vi "test capture.vi"() -> ()   [LabVIEW 2014]
uses:
  <vilib>/Utility/inputDevices.llb/joystickAcquire.vi
  <vilib>/Utility/inputDevices.llb/closeJoystick.vi
panel:
  in  "Stop All":bool=TRUE
  out "button 4":bool
  out "button 3":bool
  in  "Motor Cruise Param":T1={"X Acc (mm/s^2)"=0.3, "X Vmax (mm/s)"=0.3, "Y Acc (mm/s^2)"=0.3, "Y Vmax (mm/s)"=0.3, "Z Acc (mm/s^2)"=0.1, "Z Vmax (mm/s)"=0.1}
  out "XYZ position":sgl[](array[numeric])
  in  "Motor Limits":T2={"XMAX"=8.5, "XMIN"=-5.0, "YMAX"=6.0, "YMIN"=-6.0, "ZMAX"=1.0, "ZMIN"=-1.0}
  in  "Motor settings (X,Y)":cluster{"Vmax (mm/s)":sgl, "Acc (mm/s/s)":sgl}={"Vmax (mm/s)"=0.05, "Acc (mm/s/s)"=0.5}
  in  "Motor settings (Z)":cluster{"Vmax (mm/s)":sgl, "Acc (mm/s/s)":sgl}={"Vmax (mm/s)"=0.03, "Acc (mm/s/s)"=1.0}
  in  "Capture Exp":bool
  in  "Capture bottom":bool
  in  "Capture top":bool
  in  "Goto Bottom (F7)":bool
  in  "Goto Exp (F8)":bool
  in  "Goto Top (F6)":bool
  out "Top Dispenser":T3={"X Pos (mm)"=0.5532008, "Y Pos (mm)"=0.030929338, "Z Pos (mm)"=0.77973413} {"Y Pos (mm)" format="%.3f"; "Z Pos (mm)" format="%.3f"; "X Pos (mm)" format="%.3f"}
  out "Bottom Dispenser":T3={"X Pos (mm)"=0.600309, "Y Pos (mm)"=-1.1540928, "Z Pos (mm)"=0.7938141} {"Y Pos (mm)" format="%.3f"; "Z Pos (mm)" format="%.3f"; "X Pos (mm)" format="%.3f"}
  out "Experiment Region":T3={"X Pos (mm)"=1.4278219, "Y Pos (mm)"=-0.74810517, "Z Pos (mm)"=0.7938141} {"Y Pos (mm)" format="%.3f"; "Z Pos (mm)" format="%.3f"; "X Pos (mm)" format="%.3f"}
  out "error out":errorcluster
  in  "MG17Motor Z":refnum<k7>(container)
  in  "MG17Motor Y":refnum<k7>(container)
  in  "MG17Motor X":refnum<k7>(container)
  out "Stage Moving":bool
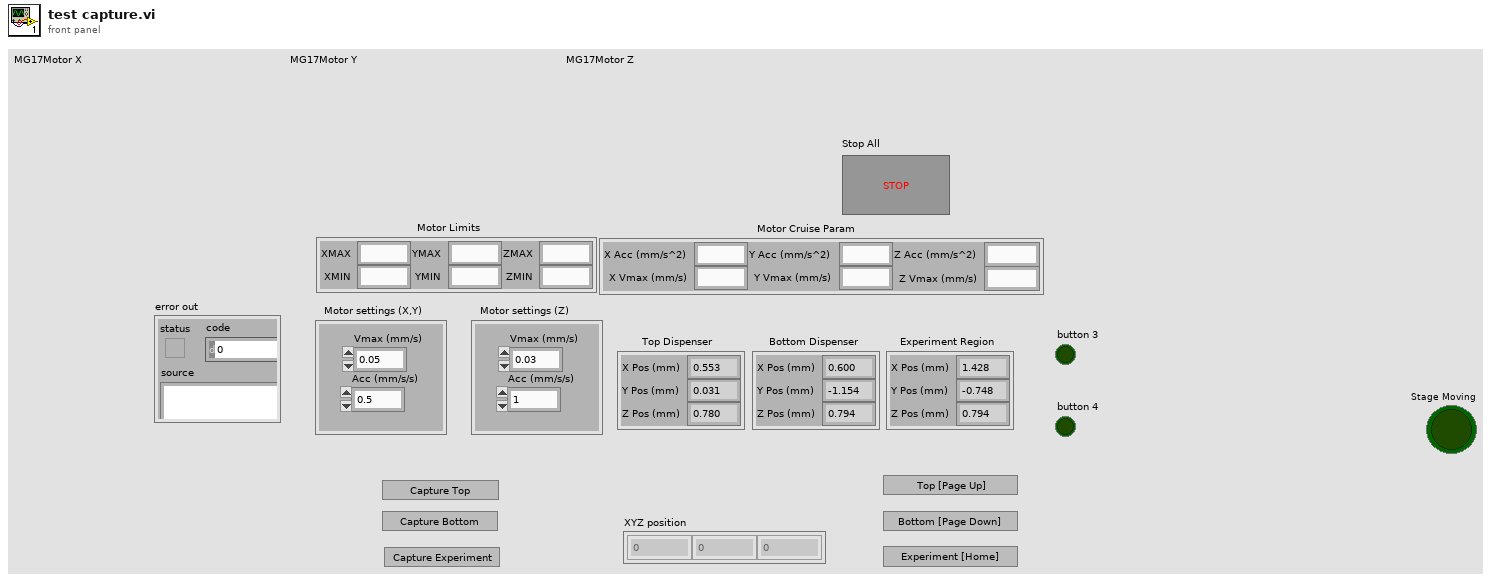
[diagram p1: front panel]
types:
  T1 = cluster{"X Acc (mm/s^2)":sgl, "X Vmax (mm/s)":sgl, "Y Acc (mm/s^2)":sgl, "Y Vmax (mm/s)":sgl, "Z Acc (mm/s^2)":sgl, "Z Vmax (mm/s)":sgl}
  T2 = cluster{"XMAX":sgl, "XMIN":sgl, "YMAX":sgl, "YMIN":sgl, "ZMAX":sgl, "ZMIN":sgl}
  T3 = cluster{"X Pos (mm)":sgl, "Y Pos (mm)":sgl, "Z Pos (mm)":sgl}
  T4 = cluster{"X axis":i32, "Y axis":i32, "Z axis":i32, "X axis rotation":i32, "Y axis rotation":i32, "Z axis rotation":i32, "U axis":i32, "V axis":i32}
  T5 = cluster{"button 1":bool, "button 2":bool, "button 3":bool, "button 4":bool, "button 5":bool, "button 6":bool, "button 7":bool, "button 8":bool, "button 9":bool, "button 10":bool, "button 11":bool, "button 12":bool, "button 13":bool, "button 14":bool, "button 15":bool, "button 16":bool, "button 17":bool, "button 18":bool, "button 19":bool, "button 20":bool, "button 21":bool, "button 22":bool, "button 23":bool, "button 24":bool, "button 25":bool, "button 26":bool, "button 27":bool, "button 28":bool, "button 29":bool, "button 30":bool, "button 31":bool, "button 32":bool}
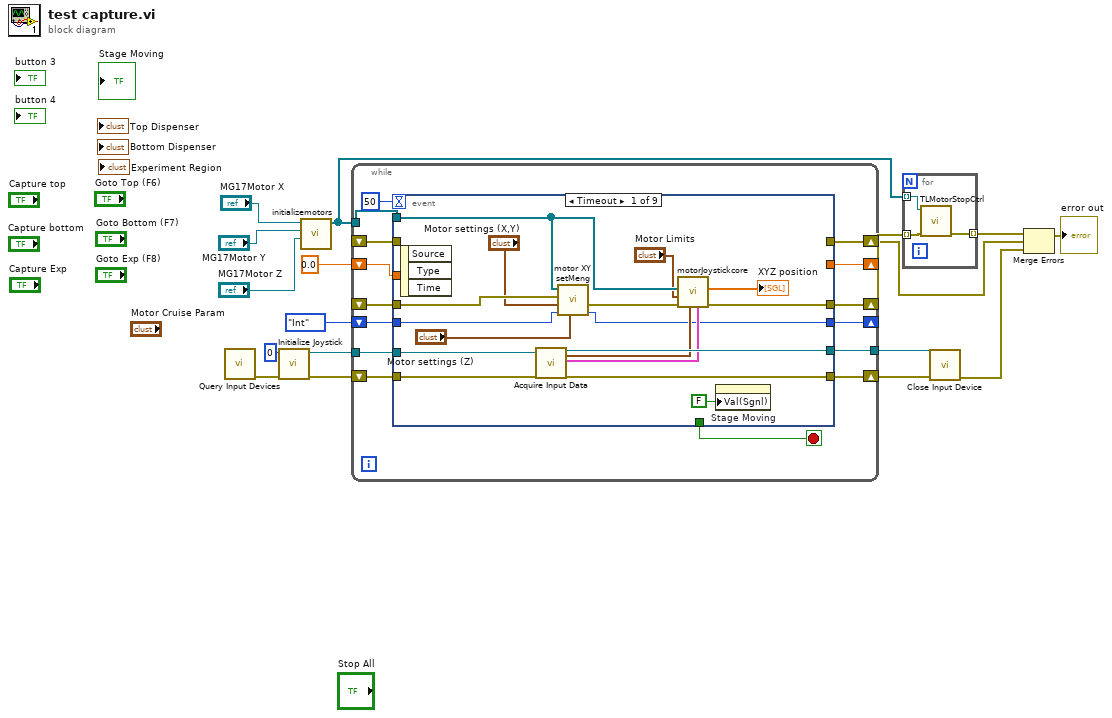
[diagram p0: block diagram]
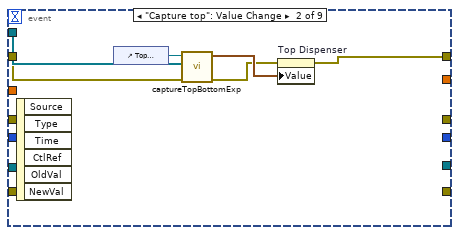
[diagram p2: hidden frame]
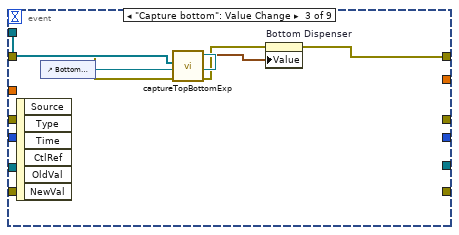
[diagram p3: hidden frame]
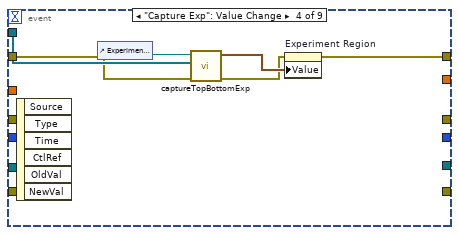
[diagram p4: hidden frame]
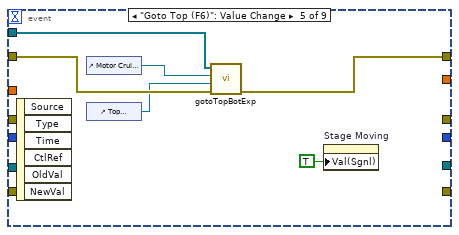
[diagram p5: hidden frame]
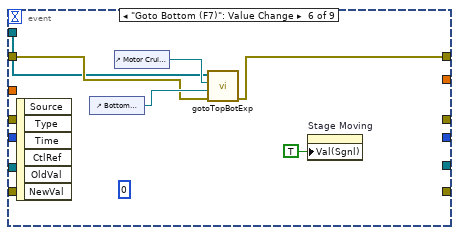
[diagram p6: hidden frame]
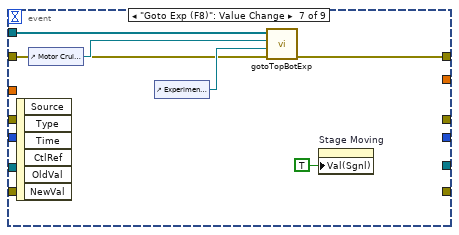
[diagram p7: hidden frame]
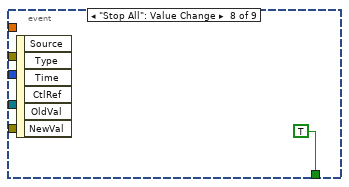
[diagram p8: hidden frame]
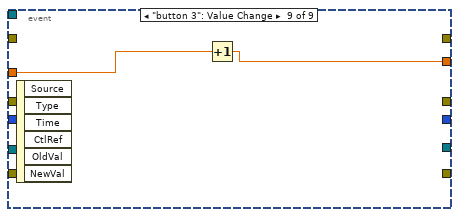
[diagram p9: hidden frame]
diagram:
  n1 = call <vilib>:"Query Input Devices.vi"() -> ("error out"=w10:errorcluster)  [unwired: 8 in, 3 out]
  n2 = call <vilib>:"Initialize Joystick.vi"("error in (no error)"=w10, "device index"=0) -> ("error out"=w7:errorcluster, "device ID"=w8:refnum<k1>)  [unwired: 8 in]
  n3 = call "initializemotors.vi"("MG17Motor Z"="MG17Motor Z", "MG17Motor Y"="MG17Motor Y", "Automation Refnum in"="MG17Motor X") -> ("Array 2"=w12:refnum<k7>[])  [unwired: 7 in, 1 out]
  n4 = while {
    tunnel: w12 -> [w32]
    shift-right: [w31] -> w2
    shift-left: _ -> [w30]
    shift-right: [w27] -> _
    shift-left: 0.0 -> [w28]
    tunnel: w8 -> [w26]
    shift-right: [w24] -> w6
    shift-left: w7 -> [w25]
    tunnel: [w23] -> w5
    shift-right: [w22] -> w3
    shift-left: _ -> [w21]
    shift-right: [w19] -> _
    shift-left: enum16{"Int", "Set"}."Int" ("Enum") -> [w20]
    stop <- w29 stop-if-true
    n5 = event shown="[0] Timeout" {
      selector: _ -> [_ _ _ _ _ _ _ _ _]
      dyn-events: _ -> [_ _ _ _ _ _ _ _ _]
      timeout: 50 -> [_ _ _ _ _ _ _ _ _]
      tunnel: w32 -> [w39 w55 w60 w67 w69 w75 w81 _ _]
      tunnel: [_ w52 w56 w62 w72 w76 w82 _ _] -> w31
      tunnel: w30 -> [_ w51 w59 w65 w73 w77 w83 _ _]
      tunnel: [_ _ _ _ _ _ _ TRUE _] -> w29
      tunnel: [_ _ _ _ _ _ _ _ w88] -> w27
      tunnel: w28 -> [_ _ _ _ _ _ _ _ w87]
      tunnel: w26 -> [w49 _ _ _ _ _ _ _ _]
      tunnel: w25 -> [w48 _ _ _ _ _ _ _ _]
      tunnel: [w47 _ _ _ _ _ _ _ _] -> w24
      tunnel: [w46 _ _ _ _ _ _ _ _] -> w23
      tunnel: [w42 _ _ _ _ _ _ _ _] -> w22
      tunnel: w21 -> [w41 _ _ _ _ _ _ _ _]
      tunnel: w20 -> [w35 _ _ _ _ _ _ _ _]
      tunnel: [w34 _ _ _ _ _ _ _ _] -> w19
      event Timeout {
        n6 = event-data() -> ()  [unwired: 1 in, 3 out]
        n7 = call-poly <vilib>:"Acquire Input Data.vi"("device ID"=w49, "error in (no error)"=w48) -> ("device ID"=w46:refnum<k1>, "axis info"=w44:T4, "button info"=w45:T5, "error out"=w47:errorcluster)  [unwired: 13 in, 1 out]
        n8 = call "motor XY setMeng.vi"("Motor settings Z"="Motor settings (Z)", "Enum in"=w35, "Motor settings (X,Y)"="Motor settings (X,Y)", "Array"=w41, "Array 2"=w39) -> ("Enum out"=w34:enum16{"Int", "Set"}, "Array 3"=w40:errorcluster[])  [unwired: 4 in, 1 out]
        n9 = call "motorJoystickcore.vi"("button info"=w45, "axis info"=w44, "error in"=w40, "Motor Limits"="Motor Limits", "Array in"=w39) -> ("error out"=w42:errorcluster[], "XYZ position"=→"XYZ position":sgl[])  [unwired: 5 in]
        n10 = property on="Stage Moving" class="Bool (strict)"("Val(Sgnl)"=FALSE ("Value (Signaling)")) -> ()  [unwired: 2 in, 2 out]
      }
      event "Capture top": Value Change {
        n11 = event-data() -> ()  [unwired: 1 in, 6 out]
        n12 = control-ref of="Top Dispenser"() -> (w50:refnum<vi>)
        n13 = call "captureTopBottomExp.vi"("error in (no error)"=w51, "Array in"=w55, "Cluster in"=w50) -> ("error out"=w53:errorcluster, "Value"=w54:T3)  [unwired: 7 in]
        n14 = property on="Top Dispenser" class="Clust (strict)"(error in=w53, "Value"=w54) -> (error out=w52:errorcluster)  [unwired: 1 in, 1 out]
      }
      event "Capture bottom": Value Change {
        n15 = event-data() -> ()  [unwired: 1 in, 6 out]
        n16 = control-ref of="Bottom Dispenser"() -> (w61:refnum<vi>)
        n17 = call "captureTopBottomExp.vi"("error in (no error)"=w59, "Array in"=w60, "Cluster in"=w61) -> ("error out"=w57:errorcluster, "Value"=w58:T3)  [unwired: 7 in]
        n18 = property on="Bottom Dispenser" class="Clust (strict)"(error in=w57, "Value"=w58) -> (error out=w56:errorcluster)  [unwired: 1 in, 1 out]
      }
      event "Capture Exp": Value Change {
        n19 = event-data() -> ()  [unwired: 1 in, 6 out]
        n20 = control-ref of="Experiment Region"() -> (w66:refnum<vi>)
        n21 = call "captureTopBottomExp.vi"("error in (no error)"=w65, "Array in"=w67, "Cluster in"=w66) -> ("error out"=w63:errorcluster, "Value"=w64:T3)  [unwired: 7 in]
        n22 = property on="Experiment Region" class="Clust (strict)"(error in=w63, "Value"=w64) -> (error out=w62:errorcluster)  [unwired: 1 in, 1 out]
      }
      event "Goto Top (F6)": Value Change {
        n23 = event-data() -> ()  [unwired: 1 in, 6 out]
        n24 = control-ref of="Motor Cruise Param"() -> (w71:refnum<vi>)
        n25 = control-ref of="Top Dispenser"() -> (w70:refnum<vi>)
        n26 = call "gotoTopBotExp.vi"("error in (no error)"=w73, "position"=w70, "motor setting"=w71, "appended array"=w69) -> ("error out"=w72:errorcluster)  [unwired: 7 in]
        n27 = property on="Stage Moving" class="Bool (strict)"("Val(Sgnl)"=TRUE ("Value (Signaling)")) -> ()  [unwired: 2 in, 2 out]
      }
      event "Goto Bottom (F7)": Value Change {
        (unwired) 0 ("lChanID")
        n28 = event-data() -> ()  [unwired: 1 in, 6 out]
        n29 = control-ref of="Bottom Dispenser"() -> (w78:refnum<vi>)
        n30 = control-ref of="Motor Cruise Param"() -> (w79:refnum<vi>)
        n31 = call "gotoTopBotExp.vi"("error in (no error)"=w77, "position"=w78, "motor setting"=w79, "appended array"=w75) -> ("error out"=w76:errorcluster)  [unwired: 7 in]
        n32 = property on="Stage Moving" class="Bool (strict)"("Val(Sgnl)"=TRUE ("Value (Signaling)")) -> ()  [unwired: 2 in, 2 out]
      }
      event "Goto Exp (F8)": Value Change {
        n33 = event-data() -> ()  [unwired: 1 in, 6 out]
        n34 = control-ref of="Motor Cruise Param"() -> (w85:refnum<vi>)
        n35 = control-ref of="Experiment Region"() -> (w84:refnum<vi>)
        n36 = call "gotoTopBotExp.vi"("error in (no error)"=w83, "position"=w84, "motor setting"=w85, "appended array"=w81) -> ("error out"=w82:errorcluster)  [unwired: 7 in]
        n37 = property on="Stage Moving" class="Bool (strict)"("Val(Sgnl)"=TRUE ("Value (Signaling)")) -> ()  [unwired: 2 in, 2 out]
      }
      event "Stop All": Value Change {
        n38 = event-data() -> ()  [unwired: 1 in, 6 out]
      }
      event "button 3": Value Change {
        n39 = event-data() -> ()  [unwired: 1 in, 6 out]
        n40 = Increment(x=w87) -> (x+1=w88:dbl)
      }
    }
  }
  n41 = for {
    tunnel: w12 -> [w91] mode=indexing
    tunnel: w3 -> [w90] mode=indexing
    tunnel: [w89] -> w14 mode=indexing
    n42 = call "TLMotorStopCtrl.vi"("Error In (No Error)"=w90, "Motor Ref"=w91) -> ("Error Out"=w89:errorcluster)  [unwired: 4 in, 1 out]
  }
  n43 = call-poly <vilib>:"Close Input Device.vi"("error in (no error)"=w6, "device ID"=w5) -> ("error out"=w1:errorcluster)  [unwired: 8 in]
  n44 = Merge Errors(w14, w2, w1) -> (→"error out":errorcluster)
